vi "Calc_Density.vi"(1 "Pres (hPa)":dbl, 2 "T (C)":dbl) -> (26 "Density (cm^-3)":dbl)   [LabVIEW 2025]
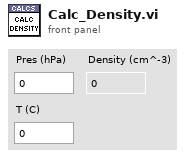
[diagram p1: front panel]
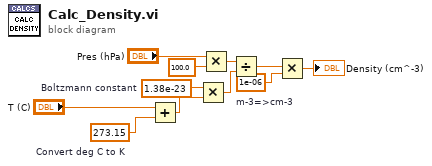
[diagram p0: block diagram]
diagram:
  w9 = 1e-06  # m-3=>cm-3
  w10 = 273.15  # Convert deg C to K
  w8 = 1.38e-23  # Boltzmann constant
  n1 = Add(x="T (C)", y=w10) -> (x+y=w7:dbl)
  n2 = Multiply(x=w8, y=w7) -> (x*y=w5:dbl)
  n3 = Multiply(x="Pres (hPa)", y=100.0) -> (x*y=w6:dbl)
  n4 = Divide(x=w6, y=w5) -> (x/y=w4:dbl)
  n5 = Multiply(x=w4, y=w9) -> (x*y=→"Density (cm^-3)":dbl)
